vi "Array_2Dto1D(Path).vi"(7 "array2D":path[][](array[path])) -> (8 "array1D":path[](array[path]))   [LabVIEW 2024]
doc: "Converts a 2D string array into a 1D string array. For example, [ [ 1 , 2 , 3 ] [ 4 , 5 , 6 ] [ 7 , 8 , 9 ] ] is converted to [ 1 , 2 , 3 , 4 , 5 , 6 , 7 , 8 , 9 ] .\n_______________________________________________________\n\nPROPRIETARY INFO:\n**********************\nThis software is the property of and contains proprietary information owned by Westinghouse Electric Company and/or its subcontractors and suppliers. It is transmitted to you in confidence and trust, and you agree to treat this software in strict accordance with the terms and conditions of the agreement under which it is provided to you. \n\n© 2011 Westinghouse Electric Company, LLC All rights reserved."
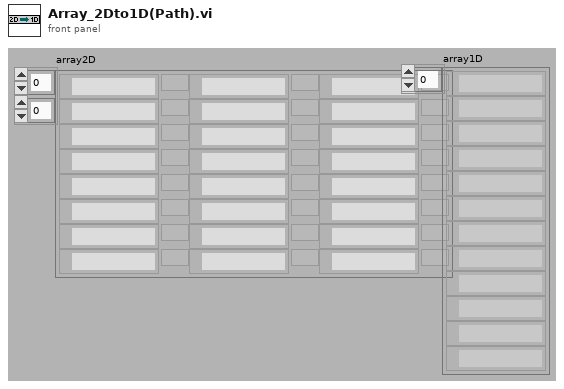
[diagram p1: front panel]
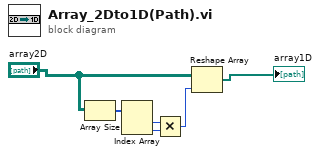
[diagram p0: block diagram]
diagram:
  n1 = Array Size(array="array2D") -> (size(s)=w6:i32[])
  n2 = Index Array(array=w6) -> (element #1=w5:i32, element #2=w4:i32)  [unwired: 2 in]
  n3 = Multiply(x=w5, y=w4) -> (x*y=w3:i32)
  n4 = Reshape Array("array2D", w3) -> (→"array1D":path[])
